vi "refresh.vi"(8 "error in (no error)":errorcluster, 10 "Engine Configuration In":refnum<class "engine configuration.lvclass">, 11 "Module Editor Node In":refnum<class "module editor node.lvclass">) -> (0 "error out":errorcluster, 2 "Engine Configuration Out":refnum<class "engine configuration.lvclass">, 3 "Module Editor Node Out":refnum<class "module editor node.lvclass">)   [LabVIEW 2013, in "PL Framework Configuration Tool.lvlib" / "module editor node.lvclass"]
uses:
  module editor node.lvclass
  <vilib>/NI/Module Execution Interface/Engine Configuration/engine configuration.lvclass
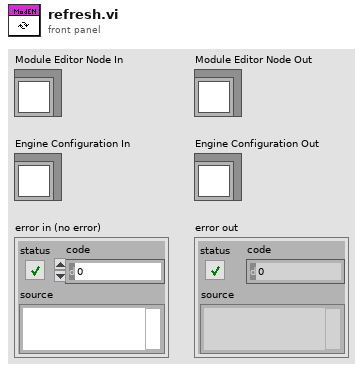
[diagram p1: front panel]
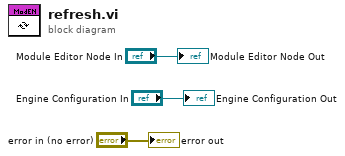
[diagram p0: block diagram]
diagram:
  "Module Editor Node Out" <- "Module Editor Node In"
  "Engine Configuration Out" <- "Engine Configuration In"
  "error out" <- "error in (no error)"
